vi "Project Directory Monitor.vi"(8 "error in (no error)":errorcluster, 9 "Control":enum16{"START", "STOP"}(ring), 11 "Editor.lvclass in":refnum<data-value>) -> (0 "error out":errorcluster, 3 "Editor.lvclass out":refnum<data-value>)   [LabVIEW 2015, in "Editor.lvclass"]
uses:
  Editor.lvclass
  Project.lvclass
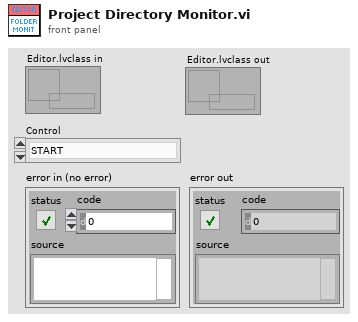
[diagram p1: front panel]
types:
  T1 = cluster{"Event":enum16{"Changed", "Created", "Deleted", "Renamed", "Error"}, "Explorer Tree":refnum<vi>, "Path":path}
  T2 = enum16{"Changed", "Created", "Deleted", "Renamed", "Error"}[]
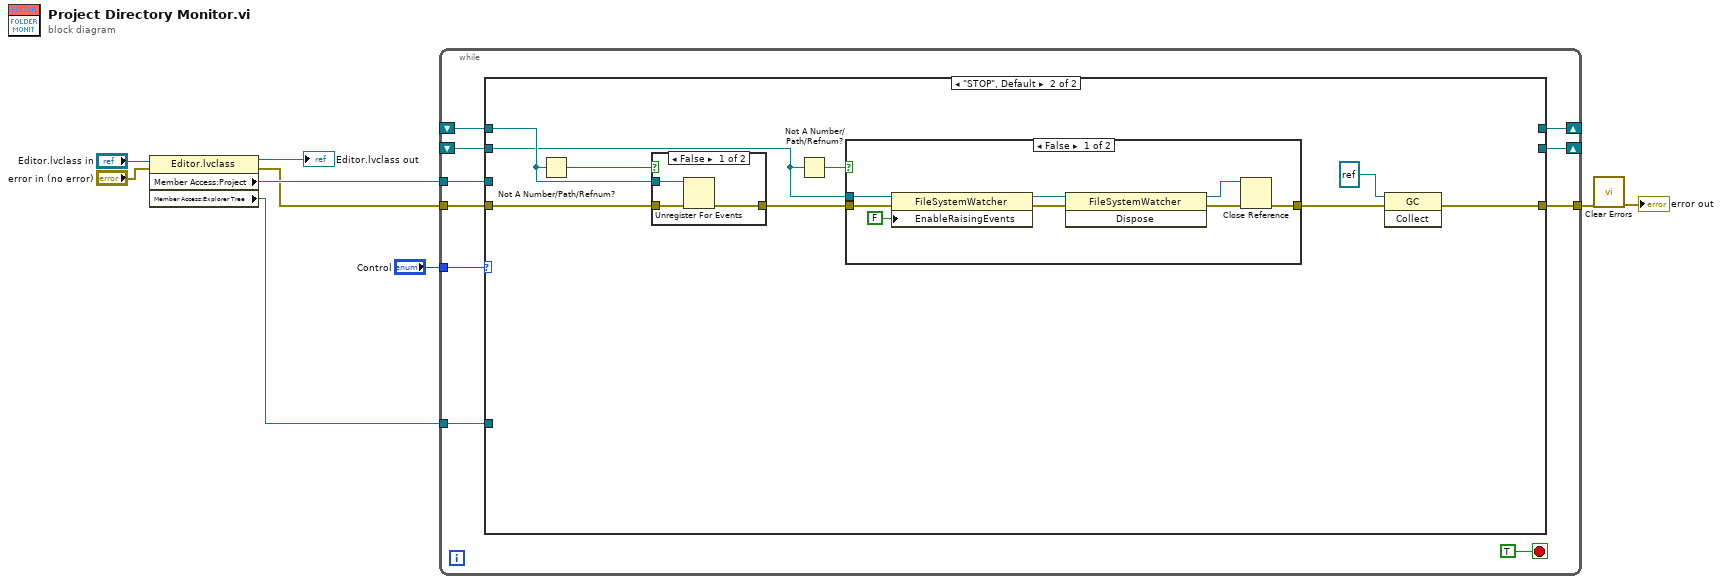
[diagram p0: block diagram]
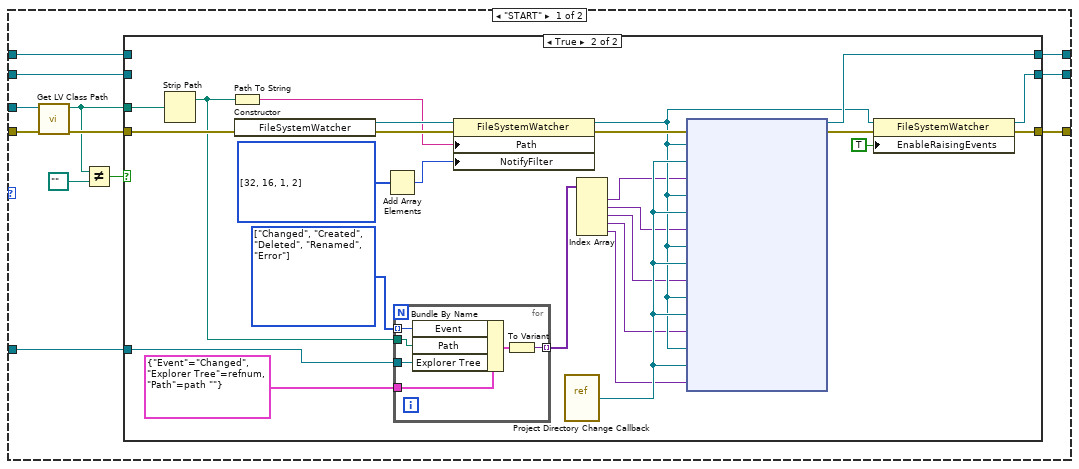
[diagram p2: hidden frame]
diagram:
  n1 = property class="Editor.lvclass"(reference="Editor.lvclass in", error in="error in (no error)") -> (reference out=→"Editor.lvclass out":refnum<data-value>, error out=w4:errorcluster, "Member Access:Project"=w6:refnum<class "Project.lvclass">, "Member Access:Explorer Tree"=w5:refnum<vi>)
  n2 = while {
    tunnel: w4 -> [w19]
    tunnel: w6 -> [w18]
    tunnel: "Control" -> [w17]
    tunnel: [w14] -> w2
    shift-right: [w13] -> _
    shift-left: _ -> [w11]
    shift-right: [w15] -> _
    shift-left: _ -> [w12]
    tunnel: w5 -> [w10]
    stop <- TRUE stop-if-true
    n3 = case shown="\"STOP\", Default" w17 {
      tunnel: w19 -> [w31 w74]
      tunnel: w18 -> [w28 _]
      tunnel: [w27 _] -> w15
      tunnel: [w26 w66] -> w14
      tunnel: [w25 _] -> w13
      tunnel: w12 -> [w20 w69]
      tunnel: w11 -> [w21 w72]
      tunnel: w10 -> [w23 _]
      frame "START" {
        n4 = call <vilib>:"Get LV Class Path.vi"("error in (no error)"=w31, "object"=w28) -> ("error out"=w29:errorcluster, "class path"=w22:path)  [unwired: 8 in]
        n5 = Not Equal?(x=w22, y=path "" ("x")) -> (x != y?=w30:bool)
        n6 = case shown="True" w30 {
          tunnel: w22 -> [_ w38]
          tunnel: w29 -> [w34 w53]
          tunnel: [w32 w51] -> w27
          tunnel: [w34 w50] -> w26
          tunnel: [w33 w49] -> w25
          tunnel: w23 -> [_ w36]
          tunnel: w21 -> [w33 _]
          tunnel: w20 -> [w32 _]
          frame False {
          }
          frame True {
            w46 = T2 [enum."Changed", enum."Created", enum."Deleted", enum."Renamed", enum."Error"] items=["Changed", "Created", "Deleted", "Renamed", "Error"]
            w57 = i32[] [32, 16, 1, 2] items=["FileName"=1, "DirectoryName"=2, "Attributes"=4, "Size"=8, "LastWrite"=16, "LastAccess"=32, "CreationTime"=64, "Security"=256]
            n7 = Strip Path(path=w38) -> (stripped path=w35:path)  [unwired: 1 out]
            n8 = Path To String(path=w35) -> (string=w37:string)
            n9 = constructor class="FileSystemWatcher"(error in=w53) -> (reference out=w59:refnum<k24>, error out=w58:errorcluster)  [unwired: 2 in, 1 out]
            n10 = Add Array Elements(numeric array=w57) -> (sum=w56:i32)
            n11 = for {
              tunnel: w46 -> [w64] mode=indexing
              tunnel: T1 {"Event"=enum."Changed", "Explorer Tree"=refnum, "Path"=path ""} -> [w65]
              tunnel: [w62] -> w44 mode=indexing
              tunnel: w36 -> [w61]
              tunnel: w35 -> [w60]
              n12 = Bundle By Name(cluster=w65, "Event"=w64, "Path"=w60, "Explorer Tree"=w61) -> (w63:T1)
              n13 = To Variant(anything=w63) -> (Variant=w62:variant)
            }
            n14 = property class="FileSystemWatcher"(reference=w59, error in=w58, "Path"=w37, "NotifyFilter"=w56) -> (reference out=w47:refnum<k24>, error out=w52:errorcluster)
            n15 = vi-ref "Project Directory Change Callback.vi"() -> ("vi reference"=w48:refnum<vi>)
            n16 = Index Array(array=w44) -> (element #1=w43:variant, element #2=w42:variant, element #3=w41:variant, element #4=w40:variant, element #5=w39:variant)  [unwired: 5 in]
            n17 = node(w52, w47, w48, w43, w47, w48, w42, w47, w48, w41, w47, w48, w40, w47, w48, w39) -> (w49:refnum<k27>, w55:errorcluster)  [unwired: 1 in]
            n18 = property class="FileSystemWatcher"(reference=w47, error in=w55, "EnableRaisingEvents"=TRUE) -> (reference out=w51:refnum<k24>, error out=w50:errorcluster)
          }
        }
      }
      frame "STOP", Default {
        n19 = Not A Number/Path/Refnum?(number/path/refnum=w72) -> (NaN/Path/Refnum?=w71:bool)
        n20 = case shown="False" w71 {
          tunnel: w74 -> [w86 w87]
          tunnel: [w85 w87] -> w73
          tunnel: w72 -> [w84 _]
          frame False {
            n21 = Unregister For Events(event registration refnum=w84, error in=w86) -> (error out=w85:errorcluster)
          }
          frame True {
          }
        }
        n22 = Not A Number/Path/Refnum?(number/path/refnum=w69) -> (NaN/Path/Refnum?=w70:bool)
        n23 = case shown="False" w70 {
          tunnel: w69 -> [w80 _]
          tunnel: w73 -> [w76 w83]
          tunnel: [w75 w83] -> w67
          frame False {
            n24 = property class="FileSystemWatcher"(reference=w80, error in=w76, "EnableRaisingEvents"=FALSE) -> (reference out=w82:refnum<k24>, error out=w79:errorcluster)
            n25 = invoke class="FileSystemWatcher" method="Dispose"(reference=w82, error in=w79) -> (reference out=w77:refnum<k24>, error out=w78:errorcluster)  [unwired: 1 in, 1 out]
            n26 = Close Reference(reference=w77, error in (no error)=w78) -> (error out=w75:errorcluster)
          }
          frame True {
          }
        }
        n27 = invoke class="GC" method="Collect"(reference=refnum<k24> refnum, error in=w67) -> (error out=w66:errorcluster)  [unwired: 1 in, 2 out]
      }
    }
  }
  n28 = call <vilib>:"Clear Errors.vi"("error in (no error)"=w2) -> ("error out"=→"error out":errorcluster)  [unwired: 5 in, 1 out]
